vi "Open skywire serial comm if not.vi"(8 "error in (no error)":errorcluster, 9 "flow control (0:none)":u16(ring) items=["None", "XON/XOFF", "RTS/CTS", "XON/XOFF & RTS/CTS", "DTR/DSR", "XON/XOFF & DTR/DSR"], 10 "Is serial open?":bool, 11 "VISA Refnum in":refnum<visa-resource-name>) -> (0 "error out":errorcluster, 3 "VISA Refnum out":refnum<visa-resource-name>)   [LabVIEW 2013]
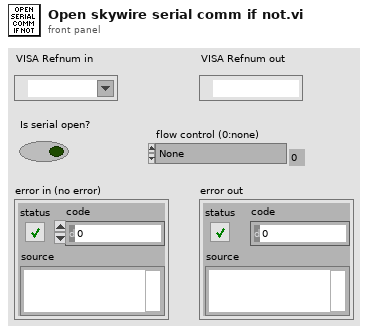
[diagram p1: front panel]
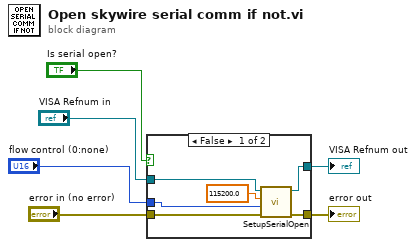
[diagram p0: block diagram]
diagram:
  n1 = case shown="False" "Is serial open?" {
    tunnel: [w8 w13] -> w5
    tunnel: "error in (no error)" -> [w11 w14]
    tunnel: [w9 w14] -> w6
    tunnel: "VISA Refnum in" -> [w12 w13]
    tunnel: "flow control (0:none)" -> [w7 _]
    frame False {
      n2 = call "SetupSerialOpen.vi"("error in (no error)"=w11, "flow control (0:none)"=w7, "Baud"=115200.0, "VISA Refnum in"=w12) -> ("error out"=w9:errorcluster, "VISA session"=w8:refnum<visa-resource-name>)  [unwired: 6 in]
    }
    frame True {
    }
  }
  "error out" <- w6
  "VISA Refnum out" <- w5
